vi "GET_Decision_about_TTL_and_Fire.vi"(8 "error in (no error)":errorcluster, 10 "Coordinates and speed":T2 {"Measurements and statistics"."Running, perc. of time" format="%05.2f"}, 11 "Settings cluster (local)":T5 {"Calibration parameters"."True frame time, s" format="%.10g"; "Calibration parameters"."Disp. calibration info"."Speed, µl per ms" format="%.3g"; "Calibration parameters"."True FPS" format="%.10g"; "Calibration parameters"."Timing calibration sw/hw" format="%.10g"; "Conditions presets array"."Specifier(s)"."Validity criteria(s)"."Validity value" min=0.0 step=0.1 format="%.2g"; "Conditions presets array"."Specifier(s)"."Value" step=1.0 format="%#.2g"; "Recording and saving"."Data post-processing"."Order" min=3 max=11 step=2; "Recording and saving"."Data post-processing"."Length" min=5 max=301 step=2; "Geometry"."Cage diameter, mm" scale=0.0..340.0}) -> (0 "error out":errorcluster, 3 "Channel output":T1)   [LabVIEW 2018, in "Tracker.lvlib"]
uses:
  Tracker.lvlib
  Controls/CTL_Settings_cluster.ctl
  Controls/CTL_Histogram_parameters.ctl
  Controls/CTL_Filter_selector.ctl
  Controls/CTL_Acquisition_speed_selector.ctl
  Controls/CTL_Segmented_plot_parameters.ctl
  Controls/CTL_IO_params_cluster.ctl
  Controls/CTL_Conditions_Array.ctl
  Controls/CTL_Conditions_Cluster.ctl
  Controls/CTL_Condition_type.ctl
  Controls/CTL_Comparison_type.ctl
  Controls/CTL_Validity_check_criteria.ctl
  Controls/CTL_Response_info.ctl
  Controls/CTL_Condition_response_type.ctl
  Controls/CTL_Reponse_port_info.ctl
  Controls/CTL_Calibration_parameters.ctl
  Controls/CTL_Dispenser_calibration_info.ctl
  Controls/CTL_Full_data_frame.ctl
  Controls/CTL_Animal_Coordinates_and_Speed.ctl
  Controls/CTL_Measurements_and_Statistics.ctl
  <extravilib>/ChannelInstances/Event Messenger-a[.](c(dbl,str))/))Channel.ctl
  <extravilib>/ChannelInstances/Event Messenger-a[.](c(dbl,str))/))Channel.vi
  <extravilib>/ChannelInstances/Event Messenger-a[.](c(dbl,str)).lvlib
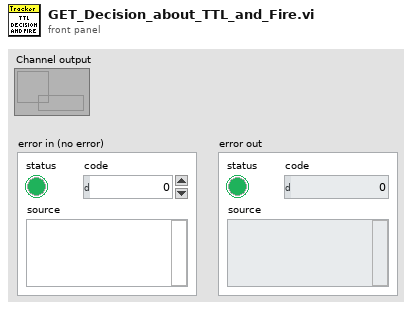
[diagram p1: front panel]
types:
  T1 = typedef "Event Messenger-a[.](c(dbl,str)).lvlib/))Channel.ctl" = refnum<queue>
  T2 = typedef "Tracker.lvlib/CTL_Full_data_frame.ctl" = cluster{"Times":cluster{"ms since ON":u32, "delta time":u32, "Frame timestamp":timestamp}, "TTLs":cluster{"TTL input":i16, "TTL output":i16}, "Animal coordinates":T3, "Magnets coords raw":cluster{"X1 raw":dbl, "Y1 raw":dbl, "X2 raw":dbl, "Y2 raw":dbl}, "Measurements and statistics":T4}
  T3 = typedef "Tracker.lvlib/CTL_Animal_Coordinates_and_Speed.ctl" = cluster{"R from center":dbl, "phi (mouse angular position in the cage)":dbl, "alpha (mouse rot. angle)":dbl, "X":dbl, "Y":dbl, "theta (from center towards mouse)":dbl, "beta (cage rot. against mouse)":dbl, "w (mouse angle to wall)":dbl, "Speed (filtered)":dbl}
  T4 = typedef "Tracker.lvlib/CTL_Measurements_and_Statistics.ctl" = cluster{"Zone #":i8, "Histogram":dbl[], "Running, perc. of time":dbl, "Run, meters":dbl, "Avg. speed":dbl}
  T5 = typedef "Tracker.lvlib/CTL_Settings_cluster.ctl" = cluster{"Defaults":cluster{"Default User":dbl, "VISA Resource Name ":string, "Histogram parameters":T6}, "Recording and saving":cluster{"Researcher name":string, "Name prefix":string, "Data post-processing":T7, "Stop at":dbl, "\"Stop at\" enabled":bool, "Default save folder path":path, "Acquisition FPS":T8}, "Geometry":T9, "IO parameters":T10, "Conditions presets array":T11, "Calibration parameters":T19, "Settings loaded OK":bool}
  T6 = typedef "Tracker.lvlib/CTL_Histogram_parameters.ctl" = cluster{"max":dbl, "min":dbl, "# bins":i32, "threshold":dbl, "thr. type":enum16{"higher accepted", "lower accepted"}}
  T7 = typedef "Tracker.lvlib/CTL_Filter_selector.ctl" = cluster{"Filter type":enum16{"None", "Savitzky-Golay"}, "Length":i32, "Order":i32}
  T8 = typedef "Tracker.lvlib/CTL_Acquisition_speed_selector.ctl" = enum16{"Max", "Optimal", "Eco"}
  T9 = typedef "Tracker.lvlib/CTL_Segmented_plot_parameters.ctl" = cluster{"Cage diameter, mm":u16, "Starting angle MIDFIELD":i16, "Starting angle BORDER":i16, "Radius, mm CENTER":u16, "Radius, mm MIDFIELD":u16, "N segments MIDFIELD":u8, "N segments BORDER":u8, "R-gap, mm":sgl, "Bridge swap":bool, "Bridge H. offset":sgl, "Bridge V. offset":sgl, "Twisted neck":bool, "Alt. magn. orientation":bool, "Sensor board size":enum16{"Small", "Large"}}
  T10 = typedef "Tracker.lvlib/CTL_IO_params_cluster.ctl" = cluster{"IO general config.":u16, "IO 1 configuration":u16, "IO 2 configuration":u16, "IO 3 configuration":u16, "IO 4 configuration":u16, "Activate ext. RS-232":u16, "IO inversion config.":u16, "Sync capability":u8}
  T11 = typedef "Tracker.lvlib/CTL_Conditions_Array.ctl" = T12[]
  T12 = typedef "Tracker.lvlib/CTL_Conditions_Cluster.ctl" = cluster{"Enabled":bool, "Name":string, "Specifier(s)":cluster{"Specifier enabled":bool, "Condition type":T13, "Comparison type":T14, "Value":dbl, "Validity criteria(s)":cluster{"V. check enabled":bool, "Criteria":T15, "Validity value":dbl}[]}[], "Response":T16, "Has been set":bool}
  T13 = typedef "Tracker.lvlib/CTL_Condition_type.ctl" = enum16{"Speed", "Zone", "Angle to wall"}
  T14 = typedef "Tracker.lvlib/CTL_Comparison_type.ctl" = enum16{"Less", "Less or Equal", "Equal", "Greater or Equal", "Greater", "Not Equal"}
  T15 = typedef "Tracker.lvlib/CTL_Validity_check_criteria.ctl" = enum16{"Running bout (seconds)", "Running bout (meters)"}
  T16 = typedef "Tracker.lvlib/CTL_Response_info.ctl" = cluster{"Response type":T17, "TTL port":T18, "TTL pulse length, ms":dbl}
  T17 = typedef "Tracker.lvlib/CTL_Condition_response_type.ctl" = enum16{"None", "Air puff", "Liquid reward"}
  T18 = typedef "Tracker.lvlib/CTL_Reponse_port_info.ctl" = enum16{"Port 1", "Port 2", "Port 3", "Port 4"}
  T19 = typedef "Tracker.lvlib/CTL_Calibration_parameters.ctl" = cluster{"Timing calibration sw/hw":dbl, "True FPS":dbl, "True frame time, s":dbl, "Disp. calibration info":T20}
  T20 = typedef "Tracker.lvlib/CTL_Dispenser_calibration_info.ctl" = cluster{"Channel":u8, "Speed, µl per ms":dbl}[]
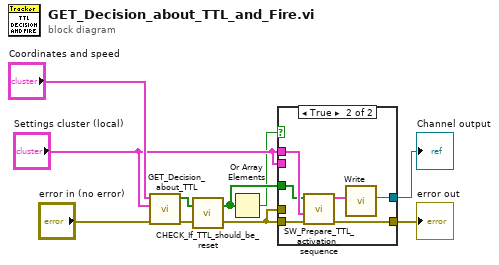
[diagram p0: block diagram]
diagram:
  n1 = call "GET_Decision_about_TTL.vi"("Error In"="error in (no error)", "Settings cluster"="Settings cluster (local)", "Current animal coordinates and stats"="Coordinates and speed") -> ("Error Out"=w6:errorcluster, "To be activated"=w5:bool[])  [unwired: 7 in]
  n2 = call "CHECK_If_TTL_should_be_reset.vi"("Error In"=w6, "To be activated in"=w5) -> ("Error Out"=w4:errorcluster, "To be activated out"=w3:bool[])
  n3 = Or Array Elements(Boolean array=w3) -> (logical OR=w2:bool)
  n4 = case shown="True" w2 {
    tunnel: [w11 w12] -> w7
    tunnel: "Settings cluster (local)" -> [_ _]
    tunnel: [_ w17] -> w1
    tunnel: w4 -> [w11 _]
    tunnel: w4 -> [_ w16]
    tunnel: "Settings cluster (local)" -> [_ w15]
    tunnel: w3 -> [_ w14]
    frame False {
    }
    frame True {
      n5 = call "SW_Prepare_TTL_activation_sequence.vi"("Error In"=w16, "Settings cluster (local)"=w15, "Rules (conditions) to activate"=w14) -> ("Error Out"=w12:errorcluster, "TTL out sequence"=w13:cluster{"Numeric":dbl, "String":string}[])  [unwired: 7 in]
      n6 = call <extravilib>:"Write.vi"("element"=w13) -> ("channel"=w17:T1)  [unwired: 9 in, 1 out]
    }
  }
  "error out" <- w7
  "Channel output" <- w1
